vi "state_detect_old.vi"() -> ()   [LabVIEW 2012]
uses:
  <vilib>/DAQmx/create/channels.llb/DAQmx Create Channel (CO-Pulse Generation-Frequency).vi
  <vilib>/DAQmx/configure/timing.llb/DAQmx Timing (Implicit).vi
  <vilib>/Analysis/NI_AALBase.lvlib
panel:
  out "Run Number":i32
  out "Fluorescence with pumping":u32
  out "Fluorescence  Without Pumping":u32
  out "x = 0?":bool
  out "Last Few":dbl[](array[numeric])
  out "Not_opt_pump_dark_runs":i32
  out "opt_pump_dark_runs":i32
  in  "Fluoresence Threshold":u32
  out "No_opt_pump_dark_run_ratio":dbl
  out "Opt_pump_Dark_run_ratio":dbl
  out "Fluorescence After":T1(graph)
  out "Fluorescence before":T1(graph)
  in  "Runs":i32
  in  "stop":bool
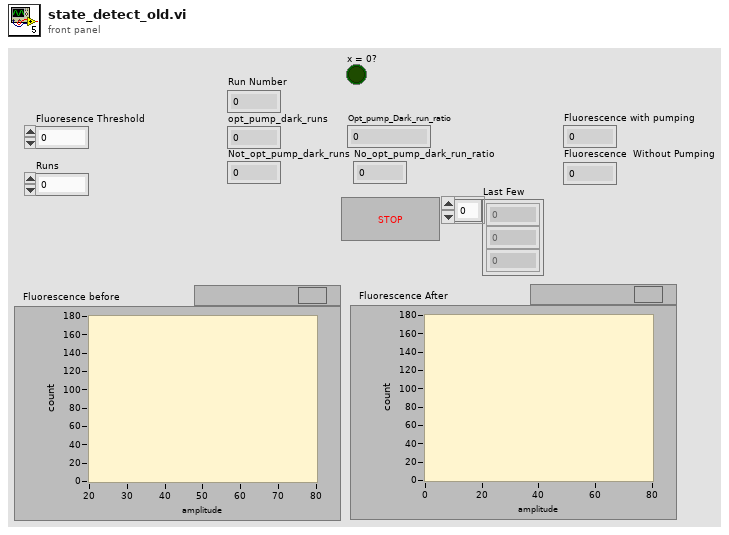
[diagram p1: front panel]
types:
  T1 = cluster{"X Values":dbl[], "Histogram: h(x)":i32[]}
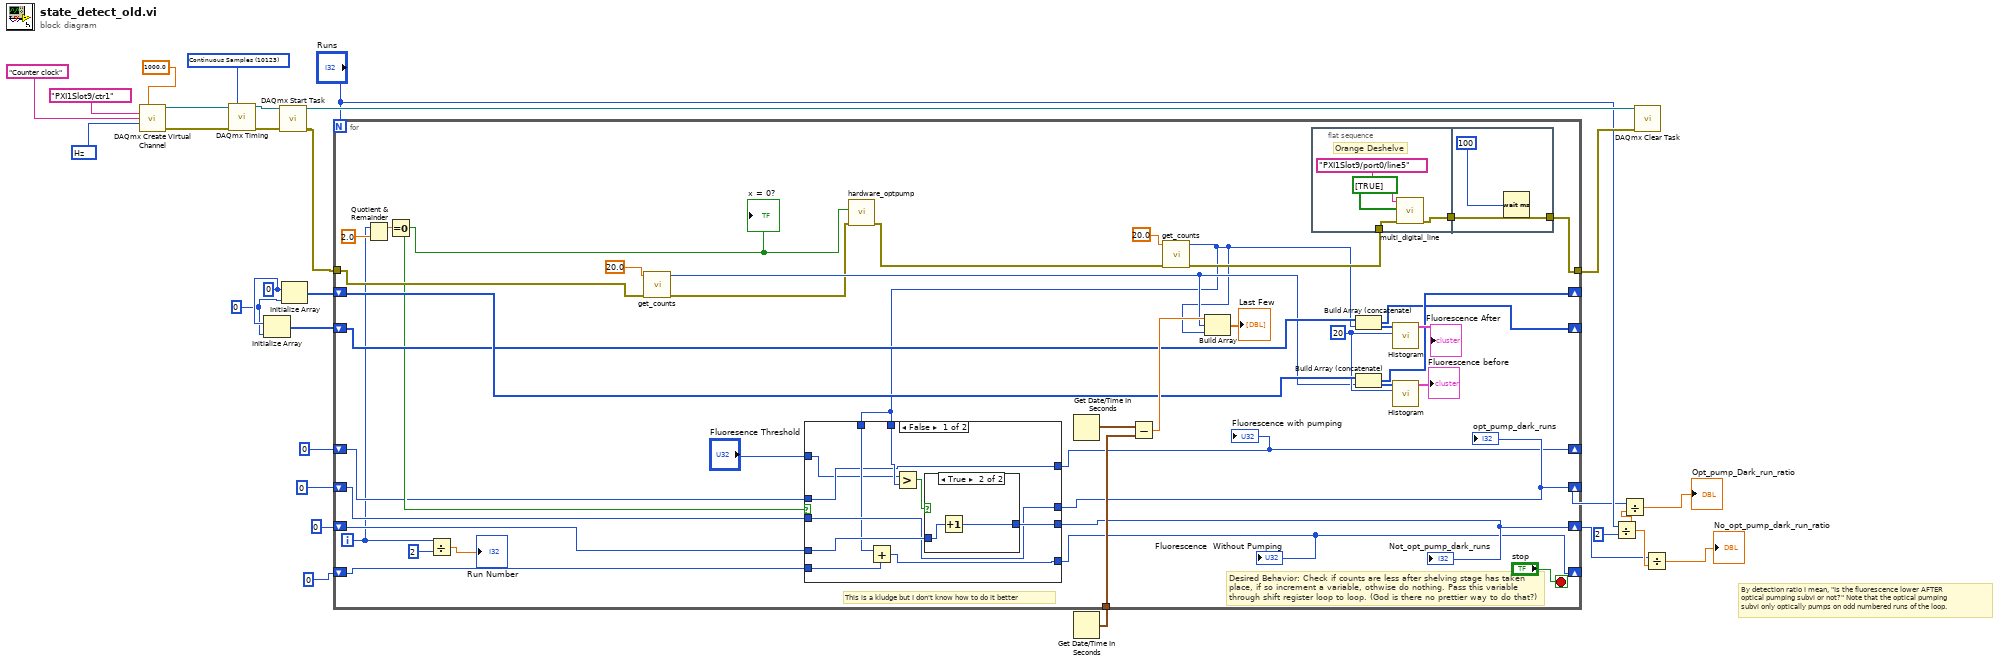
[diagram p0: block diagram]
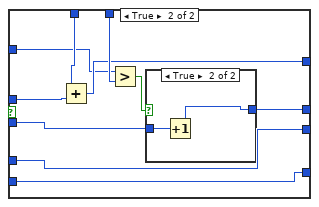
[diagram p3: hidden frame]
diagram:
  w14 = 0 ("dimension size")
  w15 = 0 ("element")
  w23 = 10123 items=["Finite Samples"=10178, "Continuous Samples"=10123, "Hardware Timed Single Point"=12522] ("sample mode")
  w28 = 10373 items=["Hz"=10373] ("units")
  # "By detection ratio I mean, \"Is the fluorescence lower AFTER\noptical pumping subvi or not?\" Note that the optical pumping\nsubvi only optically pumps on odd numbered runs of the loop."
  n1 = call-poly <vilib>:"DAQmx Create Virtual Channel.vi"("frequency"=1000.0 ("rate"), "counter"=tag "PXI1Slot9/ctr1", "name to assign"="Counter clock", "units"=w28) -> ("task out"=w27:refnum<k21>, "error out"=w26:errorcluster)  [unwired: 10 in]
  n2 = call-poly <vilib>:"DAQmx Timing.vi"("task/channels in"=w27, "sample mode"=w23, "error in"=w26) -> ("task out"=w25:refnum<k21>, "error out"=w24:errorcluster)  [unwired: 11 in]
  n3 = Initialize Array(w15, w14) -> (w12:i32[])
  n4 = call <vilib>:"DAQmx Start Task.vi"("task/channels in"=w25, "error in"=w24) -> ("task out"=w18:refnum<k21>, "error out"=w19:errorcluster)  [unwired: 12 in]
  n5 = Initialize Array(w15, w14) -> (w13:i32[])
  n6 = Get Date/Time In Seconds() -> (seconds since 1Jan1904=w17:timestamp)
  n7 = for {
    N: "Runs" -> [_]
    tunnel: w19 -> [w50]
    tunnel: w17 -> [w62]
    tunnel: [w45] -> w16
    shift-right: [w53] -> _
    shift-left: w12 -> [w58]
    shift-right: [w54] -> _
    shift-left: w13 -> [w59]
    shift-right: [w39] -> w5
    shift-left: 0 -> [w49]
    shift-right: [w38] -> w7
    shift-left: 0 -> [w48]
    shift-right: [w34] -> _
    shift-left: 0 -> [w36]
    shift-right: [w35] -> _
    shift-left: 0 -> [w37]
    i -> [w32]
    stop <- "stop" stop-if-true
    w57 = 20 ("intervals")
    # "This is a kludge but I don't know how to do it better"
    # "Desired Behavior: Check if counts are less after shelving stage has taken\nplace, if so increment a variable, othwise do nothing. Pass this variable\nthrough shift register loop to loop. (God is there no prettier way to do that?)"
    n8 = Quotient & Remainder(x=w32, y=2.0) -> (x-y*floor(x/y)=w51:dbl)  [unwired: 1 out]
    n9 = Equal To 0?(x=w51) -> (x = 0?=w43:bool)
    "x = 0?" <- w43
    n10 = Divide(x=w32, y=2) -> (x/y=→"Run Number":dbl)
    n11 = call "get_counts.vi"("error in"=w50, "Detection length (ms)"=20.0) -> ("error out"=w42:errorcluster, "Counts"=w47:u32)  [unwired: 8 in]
    n12 = call "hardware_optpump.vi"("error in"=w42, "Pump?"=w43) -> ("error out"=w41:errorcluster)  [unwired: 9 in]
    n13 = Get Date/Time In Seconds() -> (seconds since 1Jan1904=w63:timestamp)
    n14 = Subtract(x=w63, y=w62) -> (x-y=w61:dbl)
    n15 = call "get_counts.vi"("error in"=w41, "Detection length (ms)"=20.0) -> ("error out"=w46:errorcluster, "Counts"=w30:u32)  [unwired: 8 in]
    n16 = case shown="False" w43 {
      tunnel: w49 -> [w79 w91]
      tunnel: w48 -> [w77 w92]
      tunnel: w30 -> [w80 w94]
      tunnel: [w78 w91] -> w39
      tunnel: [w77 w90] -> w38
      tunnel: w30 -> [w75 w89]
      tunnel: w36 -> [w76 w88]
      tunnel: [w74 w88] -> w34
      tunnel: w37 -> [w73 w87]
      tunnel: [w73 w86] -> w35
      tunnel: "Fluoresence Threshold" -> [w72 w85]
      frame False {
        n17 = Add(x=w75, y=w76) -> (x+y=w74:u32)
        n18 = Greater?(x=w72, y=w80) -> (0:w81:bool)
        n19 = case shown="True" w81 {
          tunnel: w79 -> [w82 w84]
          tunnel: [w82 w83] -> w78
          frame False {
          }
          frame True {
            n20 = Increment(x=w84) -> (x+1=w83:i32)
          }
        }
      }
      frame True {
        n21 = Add(x=w89, y=w87) -> (x+y=w86:u32)
        n22 = Greater?(x=w85, y=w94) -> (0:w93:bool)
        n23 = case shown="True" w93 {
          tunnel: w92 -> [w95 w97]
          tunnel: [w95 w96] -> w90
          frame False {
          }
          frame True {
            n24 = Increment(x=w97) -> (x+1=w96:i32)
          }
        }
      }
    }
    "opt_pump_dark_runs" <- w38
    "Not_opt_pump_dark_runs" <- w39
    "Fluorescence with pumping" <- w35
    "Fluorescence  Without Pumping" <- w34
    n25 = Build Array(w61, w47, w30) -> (→"Last Few":dbl[])
    n26 = flat-sequence {
      tunnel: w46 -> [w69]
      tunnel: [w66] -> w44
      tunnel: [w71] -> w45
      tunnel: w44 -> [w71]
      frame #0 {
        # "Orange Deshelve"
        n27 = call "multi_digital_line.vi"("error in"=w69, "data"=bool[] [TRUE], "lines"=tag "PXI1Slot9/port0/line5" ("lines 2")) -> ("error out"=w66:errorcluster)  [unwired: 8 in]
      }
      frame #1 {
        n28 = Wait (ms)(milliseconds to wait=u32 100 ("455 Pumping Time 2")) -> ()  [unwired: 1 out]
      }
    }
    n29 = Build Array (concatenate)(w58, w30) -> (w53:u32[])
    n30 = Build Array (concatenate)(w59, w47) -> (w54:u32[])
    n31 = call <vilib>:"Histogram.vi"("intervals"=w57, "X"=w53) -> ("Histogram Graph"=→"Fluorescence After":T1)  [unwired: 6 in, 3 out]
    n32 = call <vilib>:"Histogram.vi"("intervals"=w57, "X"=w54) -> ("Histogram Graph"=→"Fluorescence before":T1)  [unwired: 6 in, 3 out]
  }
  n33 = Divide(x="Runs", y=2) -> (x/y=w6:dbl)
  n34 = Divide(x=w7, y=w6) -> (x/y=→"Opt_pump_Dark_run_ratio":dbl)
  n35 = call <vilib>:"DAQmx Clear Task.vi"("task in"=w18, "error in"=w16) -> ()  [unwired: 13 in, 1 out]
  n36 = Divide(x=w5, y=w6) -> (x/y=→"No_opt_pump_dark_run_ratio":dbl)
